vi "Latch with Reset.vi"(10 "Reset":bool, 11 "Signal In":bool) -> (3 "Signal Out":bool)   [LabVIEW 2014]
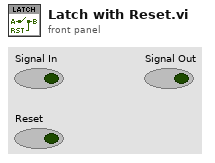
[diagram p1: front panel]
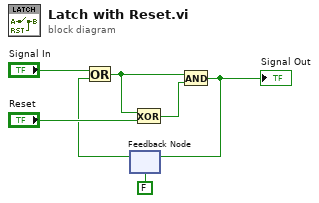
[diagram p0: block diagram]
diagram:
  n1 = feedback #1(FALSE) -> (w2:bool)
  n2 = Or(x="Signal In", y=w2) -> (x .or. y?=w5:bool)
  n3 = Exclusive Or(1:"Reset", 2:w5) -> (0:w6:bool)
  n4 = And(x=w5, y=w6) -> (x .and. y?=w7:bool)
  "Signal Out" <- w7
  n5 = feedback-in #1(w7) -> ()
